vi "controlRealTimeInChangePerPulse.vi"(7 "Set":bool, 8 "error in":errorcluster, 9 "Change in":i32, 10 "axis in":u8, 11 "connection ID":refnum<k5>) -> (0 "error out":errorcluster, 1 "Change out":i32, 2 "axis out":u8, 3 "connection ID":refnum<k5>)   [LabVIEW 2016]
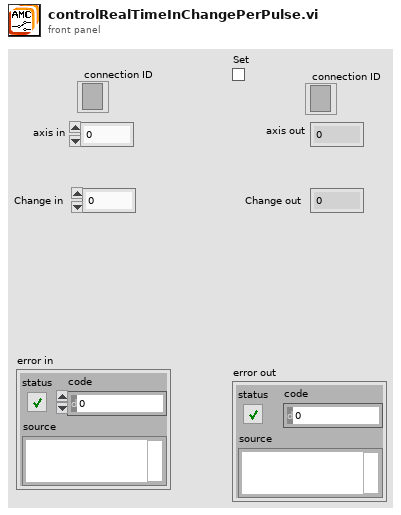
[diagram p1: front panel]
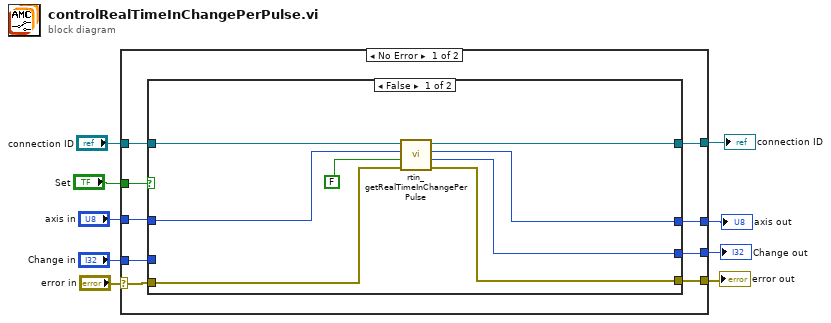
[diagram p0: block diagram]
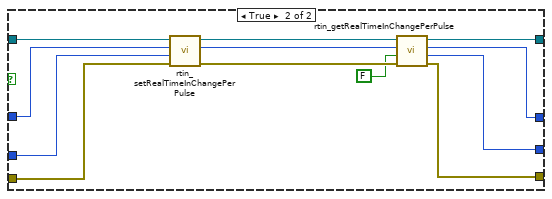
[diagram p2: hidden frame]
diagram:
  n1 = case shown="No Error" "error in" {
    selector: "error in" -> [w10 w42]
    tunnel: "axis in" -> [w17 w40]
    tunnel: [w11 w42] -> w8
    tunnel: [w13 w40] -> w7
    tunnel: "Set" -> [w18 _]
    tunnel: [w14 w39] -> w5
    tunnel: "connection ID" -> [w15 w39]
    tunnel: "Change in" -> [w16 w41]
    tunnel: [w12 w41] -> w2
    frame No Error {
      n2 = case shown="False" w18 {
        tunnel: [w25 w30] -> w14
        tunnel: w15 -> [w26 w38]
        tunnel: w17 -> [w21 w35]
        tunnel: [w24 w29] -> w13
        tunnel: [w23 w33] -> w11
        tunnel: [w19 w28] -> w12
        tunnel: w16 -> [_ w36]
        tunnel: w10 -> [w22 w37]
        frame False {
          n3 = call "rtin_getRealTimeInChangePerPulse.vi"("error in"=w22, "tempvalue"=FALSE, "axis"=w21, "connection ID"=w26) -> ("error out"=w23:errorcluster, "resolution"=w19:i32, "axis_out"=w24:i32, "connection ID"=w25:refnum<k5>)  [unwired: 4 in]
        }
        frame True {
          n4 = call "rtin_setRealTimeInChangePerPulse.vi"("error in"=w37, "resolution"=w36, "axis"=w35, "connection ID"=w38) -> ("error out"=w34:errorcluster, "axis_out"=w31:i32, "connection ID"=w32:refnum<k5>)  [unwired: 5 in]
          n5 = call "rtin_getRealTimeInChangePerPulse.vi"("error in"=w34, "tempvalue"=FALSE, "axis"=w31, "connection ID"=w32) -> ("error out"=w33:errorcluster, "resolution"=w28:i32, "axis_out"=w29:i32, "connection ID"=w30:refnum<k5>)  [unwired: 4 in]
        }
      }
    }
    frame Error {
    }
  }
  "error out" <- w8
  "axis out" <- w7
  "connection ID" <- w5
  "Change out" <- w2
